vi "Style LED Blinking.vi"() -> ()   [LabVIEW 2015]
uses:
  <vilib>/Analysis/NI_AALBase.lvlib
panel:
  out "Boolean 8":bool
  out ".not. x?":bool
  in  "Magic Nmae Disply":bool
  in  "String":string
  out "concatenated string":string
  in  "Tab Control 2":enum32{"Page 1", "Page 2"}(tab)
  in  "Boolean":bool
  in  "Boolean 2":bool
  in  "Boolean 3":bool
  in  "Boolean 4":bool
  in  "Boolean 5":bool
  in  "Boolean 6":bool
  in  "duration":dbl
  in  "Tab Control":enum32{"Page 1", "Page 2"}(tab)
  out "Array":bool[][](array[boolean])
  in  "Time_1":dbl(knob) scale=0.0..1000.0
  out "Array 2":bool[][](array[boolean])
  in  "Control Statement":bool
  out "Array 3":bool[][](array[boolean])
  in  "?":u32(knob) scale=0.0..1000.0
  out "Array 5":bool[][](array[boolean])
  in  "Time_3":u32(knob) scale=0.0..1000.0
  out "Array 4":bool[][](array[boolean])
  out "Array 6":bool[][](array[boolean])
  # "Programming Happy Dussehra"
  # "Make Own Tune Press Button to PLAY"
  # "Time_2"
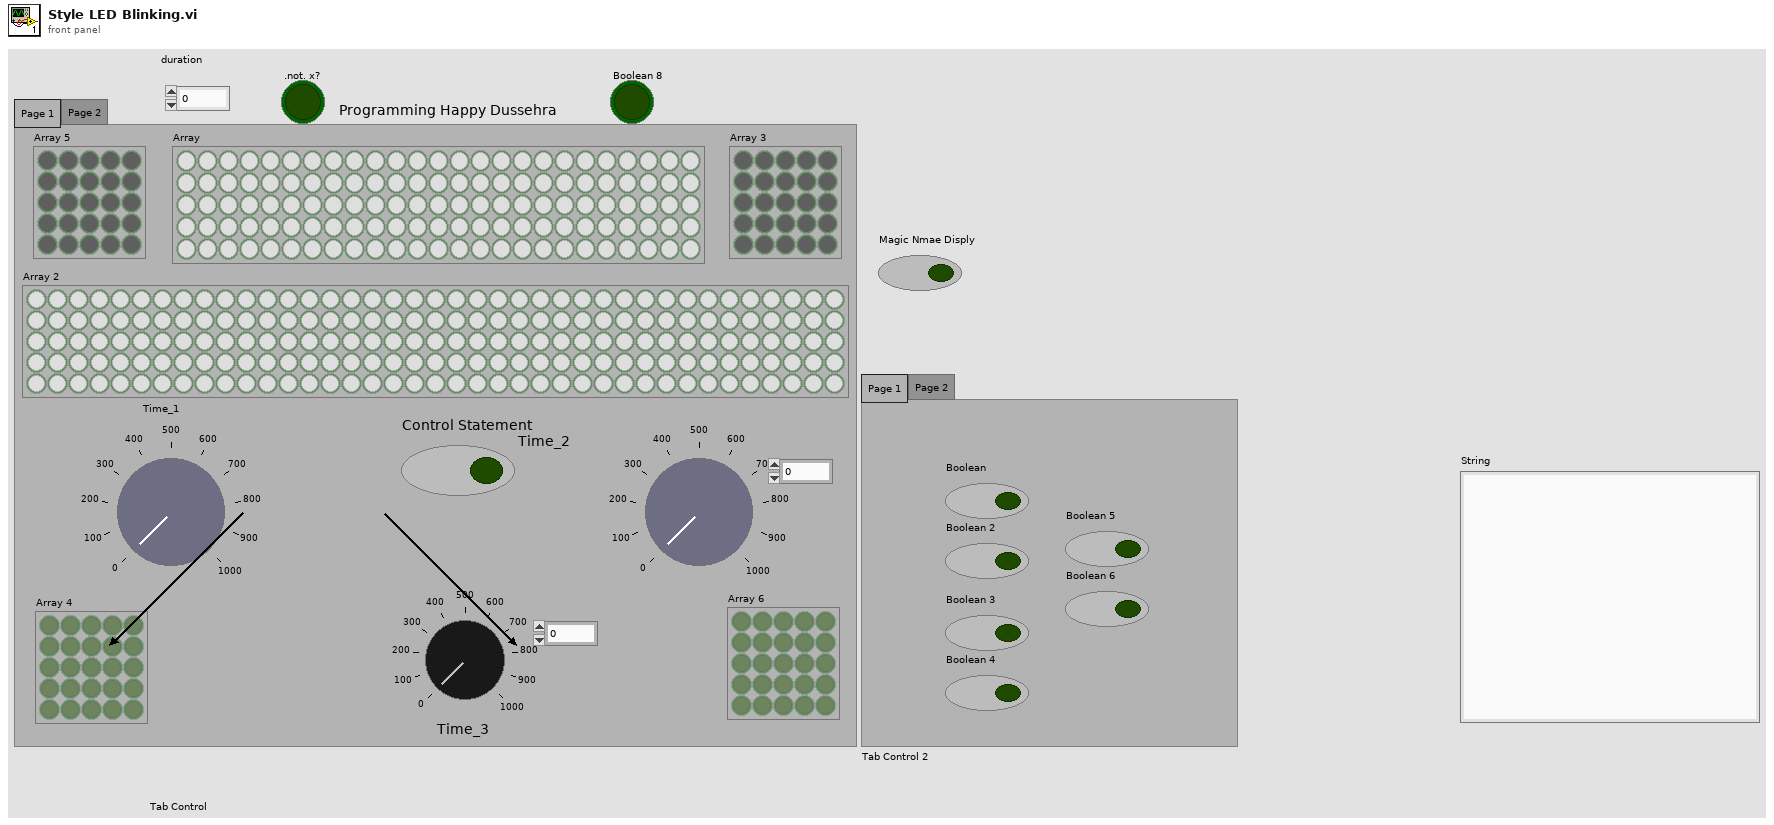
[diagram p1: front panel]
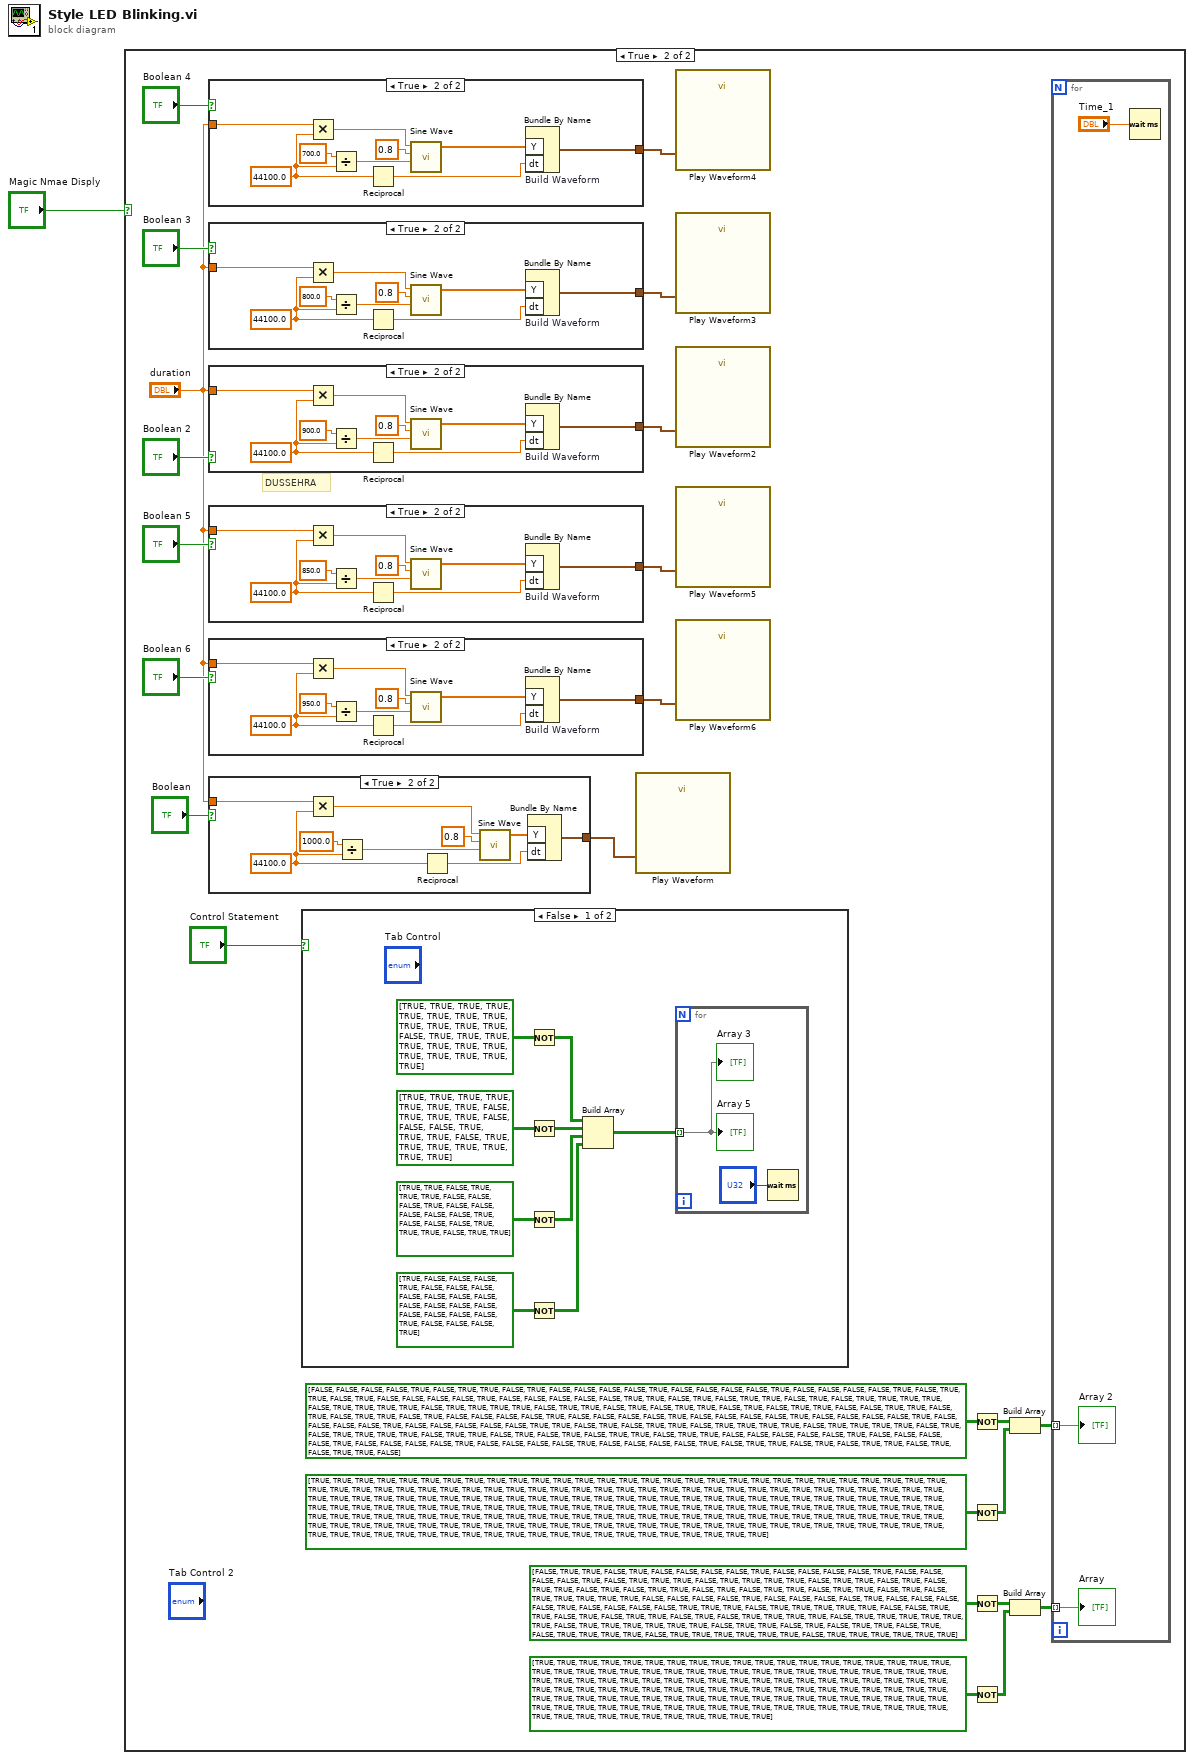
[diagram p0: block diagram]
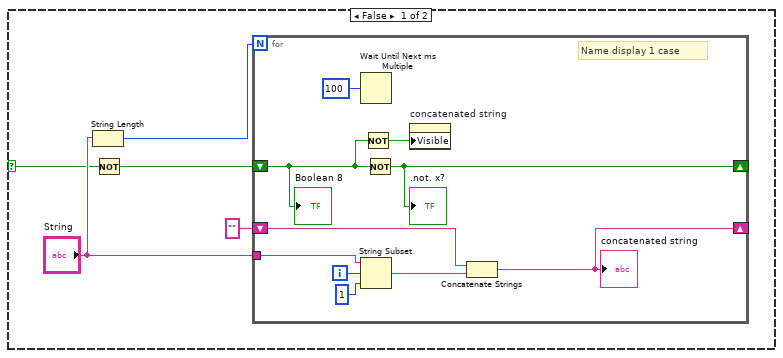
[diagram p2: hidden frame]
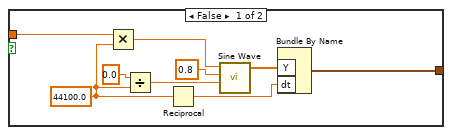
[diagram p3: hidden frame]
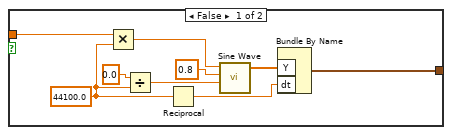
[diagram p4: hidden frame]
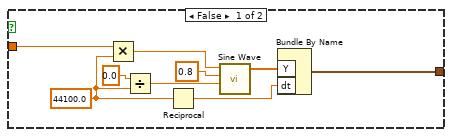
[diagram p5: hidden frame]
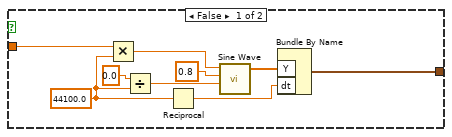
[diagram p6: hidden frame]
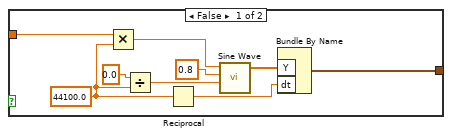
[diagram p7: hidden frame]
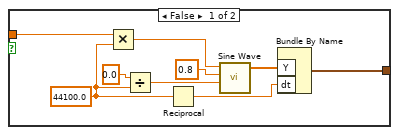
[diagram p8: hidden frame]
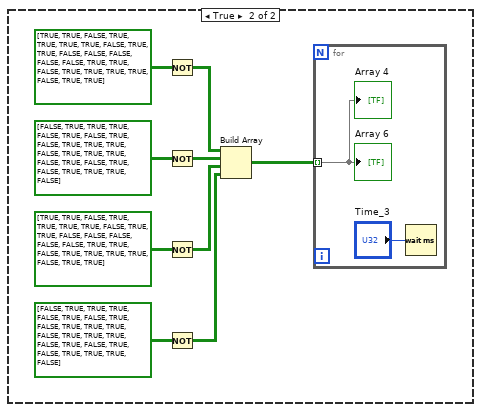
[diagram p9: hidden frame]
diagram:
  n1 = case shown="True" "Magic Nmae Disply" {
    selector: "Magic Nmae Disply" -> [w3 _]
    frame False {
      n2 = String Length(string="String") -> (length=w4:i32)
      n3 = Not(x=w3) -> (.not. x?=w2:bool)
      n4 = for {
        N: w4 -> [_]
        tunnel: "String" -> [w16]
        shift-right: [w12] -> _
        shift-left: "" -> [w11]
        shift-right: [w9] -> _
        shift-left: w2 -> [w7]
        i -> [w15]
        # "Name display 1 case"
        n5 = Wait Until Next ms Multiple(millisecond multiple=u32 100) -> ()  [unwired: 1 out]
        n6 = String Subset(string=w16, offset (0)=w15, length (rest)=1 ("length (rest)")) -> (substring=w13:string)
        n7 = Not(x=w7) -> (.not. x?=w8:bool)
        n8 = Not(x=w7) -> (.not. x?=w9:bool)
        ".not. x?" <- w9
        n9 = property on="concatenated string" class="Str"("Visible"=w8) -> ()  [unwired: 2 in, 2 out]
        n10 = Concatenate Strings "Concatenate Strings"(w11, w13) -> (w12:string)
        "concatenated string" <- w12
        "Boolean 8" <- w7
      }
    }
    frame True {
      # "DUSSEHRA"
      n11 = case shown="True" "Boolean 4" {
        tunnel: "duration" -> [w78 w88]
        tunnel: [w77 w87] -> w23
        frame False {
          w83 = 44100.0 ("fs(HZ) 3")
          n12 = Multiply(x=w78, y=w83) -> (x*y=w80:dbl)
          n13 = Divide(x=0.0 ("f(HZ) 2"), y=w83) -> (x/y=w81:dbl)
          n14 = Reciprocal(x=w83) -> (1/x=w84:dbl)
          n15 = call <vilib>:"Sine Wave.vi"("samples"=w80, "amplitude"=0.8, "frequency"=w81) -> ("sine wave"=w85:dbl[])  [unwired: 2 in, 2 out]
          n16 = Bundle By Name("Y"=w85, "dt"=w84) -> (w77:waveform(dbl))  [unwired: 1 in]
        }
        frame True {
          w92 = 44100.0 ("fs(HZ) 3")
          n17 = Multiply(x=w88, y=w92) -> (x*y=w89:dbl)
          n18 = Divide(x=700.0 ("f(HZ) 2"), y=w92) -> (x/y=w90:dbl)
          n19 = Reciprocal(x=w92) -> (1/x=w93:dbl)
          n20 = call <vilib>:"Sine Wave.vi"("samples"=w89, "amplitude"=0.8, "frequency"=w90) -> ("sine wave"=w94:dbl[])  [unwired: 2 in, 2 out]
          n21 = Bundle By Name "Build Waveform"("Y"=w94, "dt"=w93) -> (w87:waveform(dbl))  [unwired: 1 in]
        }
      }
      n22 = case shown="True" "Boolean 3" {
        tunnel: "duration" -> [w96 w106]
        tunnel: [w95 w105] -> w25
        frame False {
          w101 = 44100.0 ("fs(HZ) 3")
          n23 = Multiply(x=w96, y=w101) -> (x*y=w98:dbl)
          n24 = Divide(x=0.0 ("f(HZ) 2"), y=w101) -> (x/y=w99:dbl)
          n25 = Reciprocal(x=w101) -> (1/x=w102:dbl)
          n26 = call <vilib>:"Sine Wave.vi"("samples"=w98, "amplitude"=0.8, "frequency"=w99) -> ("sine wave"=w103:dbl[])  [unwired: 2 in, 2 out]
          n27 = Bundle By Name("Y"=w103, "dt"=w102) -> (w95:waveform(dbl))  [unwired: 1 in]
        }
        frame True {
          w110 = 44100.0 ("fs(HZ) 3")
          n28 = Multiply(x=w106, y=w110) -> (x*y=w107:dbl)
          n29 = Divide(x=800.0 ("f(HZ) 2"), y=w110) -> (x/y=w108:dbl)
          n30 = Reciprocal(x=w110) -> (1/x=w111:dbl)
          n31 = call <vilib>:"Sine Wave.vi"("samples"=w107, "amplitude"=0.8, "frequency"=w108) -> ("sine wave"=w112:dbl[])  [unwired: 2 in, 2 out]
          n32 = Bundle By Name "Build Waveform"("Y"=w112, "dt"=w111) -> (w105:waveform(dbl))  [unwired: 1 in]
        }
      }
      n33 = case shown="True" "Boolean 2" {
        tunnel: "duration" -> [w114 w124]
        tunnel: [w113 w123] -> w27
        frame False {
          w119 = 44100.0 ("fs(HZ) 3")
          n34 = Multiply(x=w114, y=w119) -> (x*y=w116:dbl)
          n35 = Divide(x=0.0 ("f(HZ) 2"), y=w119) -> (x/y=w117:dbl)
          n36 = Reciprocal(x=w119) -> (1/x=w120:dbl)
          n37 = call <vilib>:"Sine Wave.vi"("samples"=w116, "amplitude"=0.8, "frequency"=w117) -> ("sine wave"=w121:dbl[])  [unwired: 2 in, 2 out]
          n38 = Bundle By Name("Y"=w121, "dt"=w120) -> (w113:waveform(dbl))  [unwired: 1 in]
        }
        frame True {
          w128 = 44100.0 ("fs(HZ) 3")
          n39 = Multiply(x=w124, y=w128) -> (x*y=w125:dbl)
          n40 = Divide(x=900.0 ("f(HZ) 2"), y=w128) -> (x/y=w126:dbl)
          n41 = Reciprocal(x=w128) -> (1/x=w129:dbl)
          n42 = call <vilib>:"Sine Wave.vi"("samples"=w125, "amplitude"=0.8, "frequency"=w126) -> ("sine wave"=w130:dbl[])  [unwired: 2 in, 2 out]
          n43 = Bundle By Name "Build Waveform"("Y"=w130, "dt"=w129) -> (w123:waveform(dbl))  [unwired: 1 in]
        }
      }
      n44 = case shown="True" "Boolean 5" {
        tunnel: "duration" -> [w60 w70]
        tunnel: [w59 w69] -> w21
        frame False {
          w65 = 44100.0 ("fs(HZ) 3")
          n45 = Multiply(x=w60, y=w65) -> (x*y=w62:dbl)
          n46 = Divide(x=0.0 ("f(HZ) 2"), y=w65) -> (x/y=w63:dbl)
          n47 = Reciprocal(x=w65) -> (1/x=w66:dbl)
          n48 = call <vilib>:"Sine Wave.vi"("samples"=w62, "amplitude"=0.8, "frequency"=w63) -> ("sine wave"=w67:dbl[])  [unwired: 2 in, 2 out]
          n49 = Bundle By Name("Y"=w67, "dt"=w66) -> (w59:waveform(dbl))  [unwired: 1 in]
        }
        frame True {
          w74 = 44100.0 ("fs(HZ) 3")
          n50 = Multiply(x=w70, y=w74) -> (x*y=w71:dbl)
          n51 = Divide(x=850.0 ("f(HZ) 2"), y=w74) -> (x/y=w72:dbl)
          n52 = Reciprocal(x=w74) -> (1/x=w75:dbl)
          n53 = call <vilib>:"Sine Wave.vi"("samples"=w71, "amplitude"=0.8, "frequency"=w72) -> ("sine wave"=w76:dbl[])  [unwired: 2 in, 2 out]
          n54 = Bundle By Name "Build Waveform"("Y"=w76, "dt"=w75) -> (w69:waveform(dbl))  [unwired: 1 in]
        }
      }
      n55 = case shown="True" "Boolean 6" {
        tunnel: "duration" -> [w42 w52]
        tunnel: [w41 w51] -> w19
        frame False {
          w47 = 44100.0 ("fs(HZ) 3")
          n56 = Multiply(x=w42, y=w47) -> (x*y=w44:dbl)
          n57 = Divide(x=0.0 ("f(HZ) 2"), y=w47) -> (x/y=w45:dbl)
          n58 = Reciprocal(x=w47) -> (1/x=w48:dbl)
          n59 = call <vilib>:"Sine Wave.vi"("samples"=w44, "amplitude"=0.8, "frequency"=w45) -> ("sine wave"=w49:dbl[])  [unwired: 2 in, 2 out]
          n60 = Bundle By Name("Y"=w49, "dt"=w48) -> (w41:waveform(dbl))  [unwired: 1 in]
        }
        frame True {
          w56 = 44100.0 ("fs(HZ) 3")
          n61 = Multiply(x=w52, y=w56) -> (x*y=w53:dbl)
          n62 = Divide(x=950.0 ("f(HZ) 2"), y=w56) -> (x/y=w54:dbl)
          n63 = Reciprocal(x=w56) -> (1/x=w57:dbl)
          n64 = call <vilib>:"Sine Wave.vi"("samples"=w53, "amplitude"=0.8, "frequency"=w54) -> ("sine wave"=w58:dbl[])  [unwired: 2 in, 2 out]
          n65 = Bundle By Name "Build Waveform"("Y"=w58, "dt"=w57) -> (w51:waveform(dbl))  [unwired: 1 in]
        }
      }
      n66 = case shown="True" "Boolean" {
        tunnel: "duration" -> [w132 w142]
        tunnel: [w131 w141] -> w17
        frame False {
          w137 = 44100.0 ("fs(HZ) 3")
          n67 = Multiply(x=w132, y=w137) -> (x*y=w134:dbl)
          n68 = Divide(x=0.0 ("f(HZ) 2"), y=w137) -> (x/y=w135:dbl)
          n69 = Reciprocal(x=w137) -> (1/x=w138:dbl)
          n70 = call <vilib>:"Sine Wave.vi"("samples"=w134, "amplitude"=0.8, "frequency"=w135) -> ("sine wave"=w139:dbl[])  [unwired: 2 in, 2 out]
          n71 = Bundle By Name("Y"=w139, "dt"=w138) -> (w131:waveform(dbl))  [unwired: 1 in]
        }
        frame True {
          w146 = 44100.0 ("fs(HZ) 3")
          n72 = Multiply(x=w142, y=w146) -> (x*y=w143:dbl)
          n73 = Divide(x=1000.0 ("f(HZ) 2"), y=w146) -> (x/y=w144:dbl)
          n74 = Reciprocal(x=w146) -> (1/x=w147:dbl)
          n75 = call <vilib>:"Sine Wave.vi"("samples"=w143, "amplitude"=0.8, "frequency"=w144) -> ("sine wave"=w148:dbl[])  [unwired: 2 in, 2 out]
          n76 = Bundle By Name("Y"=w148, "dt"=w147) -> (w141:waveform(dbl))  [unwired: 1 in]
        }
      }
      n77 = case shown="False" "Control Statement" {
        frame False {
          n78 = Not(x=bool[][] [[TRUE, TRUE, TRUE, TRUE, TRUE], [TRUE, TRUE, TRUE, TRUE, TRUE], [TRUE, TRUE, FALSE, TRUE, TRUE], [TRUE, TRUE, TRUE, TRUE, TRUE], [TRUE, TRUE, TRUE, TRUE, TRUE]]) -> (.not. x?=w153:bool[][])
          n79 = Not(x=bool[][] [[TRUE, TRUE, TRUE, TRUE, TRUE], [TRUE, TRUE, FALSE, TRUE, TRUE], [TRUE, FALSE, FALSE, FALSE, TRUE], [TRUE, TRUE, FALSE, TRUE, TRUE], [TRUE, TRUE, TRUE, TRUE, TRUE]]) -> (.not. x?=w152:bool[][])
          n80 = Not(x=bool[][] [[TRUE, TRUE, FALSE, TRUE, TRUE], [TRUE, FALSE, FALSE, FALSE, TRUE], [FALSE, FALSE, FALSE, FALSE, FALSE], [TRUE, FALSE, FALSE, FALSE, TRUE], [TRUE, TRUE, FALSE, TRUE, TRUE]]) -> (.not. x?=w151:bool[][])
          n81 = Not(x=bool[][] [[TRUE, FALSE, FALSE, FALSE, TRUE], [FALSE, FALSE, FALSE, FALSE, FALSE], [FALSE, FALSE, FALSE, FALSE, FALSE], [FALSE, FALSE, FALSE, FALSE, FALSE], [TRUE, FALSE, FALSE, FALSE, TRUE]]) -> (.not. x?=w150:bool[][])
          n82 = Build Array "Build Array"(w153, w152, w151, w150) -> (w149:bool[][][])
          n83 = for {
            tunnel: w149 -> [w158] mode=indexing
            n84 = Wait (ms)(milliseconds to wait="?") -> ()  [unwired: 1 out]
            "Array 3" <- w158
            "Array 5" <- w158
          }
        }
        frame True {
          n85 = Not(x=bool[][] [[TRUE, TRUE, FALSE, TRUE, TRUE], [TRUE, TRUE, FALSE, TRUE, TRUE], [FALSE, FALSE, FALSE, FALSE, FALSE], [TRUE, TRUE, FALSE, TRUE, TRUE], [TRUE, TRUE, FALSE, TRUE, TRUE]]) -> (.not. x?=w164:bool[][])
          n86 = Not(x=bool[][] [[FALSE, TRUE, TRUE, TRUE, FALSE], [TRUE, FALSE, TRUE, FALSE, TRUE], [TRUE, TRUE, FALSE, TRUE, TRUE], [TRUE, FALSE, TRUE, FALSE, TRUE], [FALSE, TRUE, TRUE, TRUE, FALSE]]) -> (.not. x?=w163:bool[][])
          n87 = Not(x=bool[][] [[TRUE, TRUE, FALSE, TRUE, TRUE], [TRUE, TRUE, FALSE, TRUE, TRUE], [FALSE, FALSE, FALSE, FALSE, FALSE], [TRUE, TRUE, FALSE, TRUE, TRUE], [TRUE, TRUE, FALSE, TRUE, TRUE]]) -> (.not. x?=w162:bool[][])
          n88 = Not(x=bool[][] [[FALSE, TRUE, TRUE, TRUE, FALSE], [TRUE, FALSE, TRUE, FALSE, TRUE], [TRUE, TRUE, FALSE, TRUE, TRUE], [TRUE, FALSE, TRUE, FALSE, TRUE], [FALSE, TRUE, TRUE, TRUE, FALSE]]) -> (.not. x?=w161:bool[][])
          n89 = Build Array "Build Array"(w164, w163, w162, w161) -> (w160:bool[][][])
          n90 = for {
            tunnel: w160 -> [w169] mode=indexing
            n91 = Wait (ms)(milliseconds to wait="Time_3") -> ()  [unwired: 1 out]
            "Array 4" <- w169
            "Array 6" <- w169
          }
        }
      }
      n92 = call "Play Waveform"("Data"=w17) -> ()  [unwired: 18 in, 1 out]
      n93 = call "Play Waveform4"("Data"=w23) -> ()  [unwired: 18 in, 1 out]
      n94 = call "Play Waveform3"("Data"=w25) -> ()  [unwired: 18 in, 1 out]
      n95 = call "Play Waveform2"("Data"=w27) -> ()  [unwired: 18 in, 1 out]
      n96 = call "Play Waveform5"("Data"=w21) -> ()  [unwired: 18 in, 1 out]
      n97 = call "Play Waveform6"("Data"=w19) -> ()  [unwired: 18 in, 1 out]
      n98 = Not(x=bool[][] [[FALSE, FALSE, FALSE, FALSE, TRUE, FALSE, TRUE, TRUE, FALSE, TRUE, FALSE, FALSE, FALSE, FALSE, TRUE, FALSE, FALSE, FALSE, FALSE, TRUE, FALSE, FALSE, FALSE, FALSE, TRUE, FALSE, TRUE, TRUE, FALSE, TRUE, FALSE, FALSE, FALSE, FALSE, TRUE, FALSE, FALSE, FALSE, FALSE], [FALSE, TRUE, TRUE, FALSE, TRUE, FALSE, TRUE, TRUE, FALSE, TRUE, FALSE, TRUE, TRUE, TRUE, TRUE, FALSE, TRUE, TRUE, TRUE, TRUE, FALSE, TRUE, TRUE, TRUE, TRUE, FALSE, TRUE, TRUE, FALSE, TRUE, FALSE, TRUE, TRUE, FALSE, TRUE, FALSE, TRUE, TRUE, FALSE], [FALSE, TRUE, TRUE, FALSE, TRUE, FALSE, TRUE, TRUE, FALSE, TRUE, FALSE, FALSE, FALSE, FALSE, TRUE, FALSE, FALSE, FALSE, FALSE, TRUE, FALSE, FALSE, FALSE, FALSE, TRUE, FALSE, FALSE, FALSE, FALSE, TRUE, FALSE, FALSE, FALSE, FALSE, TRUE, FALSE, FALSE, FALSE, FALSE], [FALSE, TRUE, TRUE, FALSE, TRUE, FALSE, TRUE, TRUE, FALSE, TRUE, TRUE, TRUE, TRUE, FALSE, TRUE, TRUE, TRUE, TRUE, FALSE, TRUE, FALSE, TRUE, TRUE, TRUE, TRUE, FALSE, TRUE, TRUE, FALSE, TRUE, FALSE, TRUE, FALSE, TRUE, TRUE, FALSE, TRUE, TRUE, FALSE], [FALSE, FALSE, FALSE, FALSE, TRUE, FALSE, FALSE, FALSE, FALSE, TRUE, FALSE, FALSE, FALSE, FALSE, TRUE, FALSE, FALSE, FALSE, FALSE, TRUE, FALSE, FALSE, FALSE, FALSE, TRUE, FALSE, TRUE, TRUE, FALSE, TRUE, FALSE, TRUE, TRUE, FALSE, TRUE, FALSE, TRUE, TRUE, FALSE]]) -> (.not. x?=w33:bool[][])
      n99 = Not(x=bool[][] [[TRUE, TRUE, TRUE, TRUE, TRUE, TRUE, TRUE, TRUE, TRUE, TRUE, TRUE, TRUE, TRUE, TRUE, TRUE, TRUE, TRUE, TRUE, TRUE, TRUE, TRUE, TRUE, TRUE, TRUE, TRUE, TRUE, TRUE, TRUE, TRUE, TRUE, TRUE, TRUE, TRUE, TRUE, TRUE, TRUE, TRUE, TRUE, TRUE], [TRUE, TRUE, TRUE, TRUE, TRUE, TRUE, TRUE, TRUE, TRUE, TRUE, TRUE, TRUE, TRUE, TRUE, TRUE, TRUE, TRUE, TRUE, TRUE, TRUE, TRUE, TRUE, TRUE, TRUE, TRUE, TRUE, TRUE, TRUE, TRUE, TRUE, TRUE, TRUE, TRUE, TRUE, TRUE, TRUE, TRUE, TRUE, TRUE], [TRUE, TRUE, TRUE, TRUE, TRUE, TRUE, TRUE, TRUE, TRUE, TRUE, TRUE, TRUE, TRUE, TRUE, TRUE, TRUE, TRUE, TRUE, TRUE, TRUE, TRUE, TRUE, TRUE, TRUE, TRUE, TRUE, TRUE, TRUE, TRUE, TRUE, TRUE, TRUE, TRUE, TRUE, TRUE, TRUE, TRUE, TRUE, TRUE], [TRUE, TRUE, TRUE, TRUE, TRUE, TRUE, TRUE, TRUE, TRUE, TRUE, TRUE, TRUE, TRUE, TRUE, TRUE, TRUE, TRUE, TRUE, TRUE, TRUE, TRUE, TRUE, TRUE, TRUE, TRUE, TRUE, TRUE, TRUE, TRUE, TRUE, TRUE, TRUE, TRUE, TRUE, TRUE, TRUE, TRUE, TRUE, TRUE], [TRUE, TRUE, TRUE, TRUE, TRUE, TRUE, TRUE, TRUE, TRUE, TRUE, TRUE, TRUE, TRUE, TRUE, TRUE, TRUE, TRUE, TRUE, TRUE, TRUE, TRUE, TRUE, TRUE, TRUE, TRUE, TRUE, TRUE, TRUE, TRUE, TRUE, TRUE, TRUE, TRUE, TRUE, TRUE, TRUE, TRUE, TRUE, TRUE]]) -> (.not. x?=w32:bool[][])
      n100 = Not(x=bool[][] [[FALSE, TRUE, TRUE, FALSE, TRUE, FALSE, FALSE, FALSE, FALSE, TRUE, FALSE, FALSE, FALSE, FALSE, TRUE, FALSE, FALSE, FALSE, FALSE, TRUE, FALSE, TRUE, TRUE, TRUE, FALSE, TRUE, TRUE, TRUE, TRUE], [FALSE, TRUE, TRUE, FALSE, TRUE, FALSE, TRUE, TRUE, FALSE, TRUE, FALSE, TRUE, TRUE, FALSE, TRUE, FALSE, TRUE, TRUE, FALSE, TRUE, TRUE, FALSE, TRUE, FALSE, TRUE, TRUE, TRUE, TRUE, TRUE], [FALSE, FALSE, FALSE, FALSE, TRUE, FALSE, FALSE, FALSE, FALSE, TRUE, FALSE, FALSE, FALSE, FALSE, TRUE, FALSE, FALSE, FALSE, FALSE, TRUE, TRUE, TRUE, FALSE, TRUE, TRUE, TRUE, TRUE, TRUE, FALSE], [FALSE, TRUE, TRUE, FALSE, TRUE, FALSE, TRUE, TRUE, FALSE, TRUE, FALSE, TRUE, TRUE, TRUE, TRUE, FALSE, TRUE, TRUE, TRUE, TRUE, TRUE, TRUE, FALSE, TRUE, TRUE, TRUE, TRUE, TRUE, TRUE], [FALSE, TRUE, TRUE, FALSE, TRUE, FALSE, TRUE, TRUE, FALSE, TRUE, FALSE, TRUE, TRUE, TRUE, TRUE, FALSE, TRUE, TRUE, TRUE, TRUE, TRUE, TRUE, FALSE, TRUE, TRUE, TRUE, TRUE, TRUE, TRUE]]) -> (.not. x?=w38:bool[][])
      n101 = Not(x=bool[][] [[TRUE, TRUE, TRUE, TRUE, TRUE, TRUE, TRUE, TRUE, TRUE, TRUE, TRUE, TRUE, TRUE, TRUE, TRUE, TRUE, TRUE, TRUE, TRUE, TRUE, TRUE, TRUE, TRUE, TRUE, TRUE], [TRUE, TRUE, TRUE, TRUE, TRUE, TRUE, TRUE, TRUE, TRUE, TRUE, TRUE, TRUE, TRUE, TRUE, TRUE, TRUE, TRUE, TRUE, TRUE, TRUE, TRUE, TRUE, TRUE, TRUE, TRUE], [TRUE, TRUE, TRUE, TRUE, TRUE, TRUE, TRUE, TRUE, TRUE, TRUE, TRUE, TRUE, TRUE, TRUE, TRUE, TRUE, TRUE, TRUE, TRUE, TRUE, TRUE, TRUE, TRUE, TRUE, TRUE], [TRUE, TRUE, TRUE, TRUE, TRUE, TRUE, TRUE, TRUE, TRUE, TRUE, TRUE, TRUE, TRUE, TRUE, TRUE, TRUE, TRUE, TRUE, TRUE, TRUE, TRUE, TRUE, TRUE, TRUE, TRUE], [TRUE, TRUE, TRUE, TRUE, TRUE, TRUE, TRUE, TRUE, TRUE, TRUE, TRUE, TRUE, TRUE, TRUE, TRUE, TRUE, TRUE, TRUE, TRUE, TRUE, TRUE, TRUE, TRUE, TRUE, TRUE]]) -> (.not. x?=w36:bool[][])
      n102 = Build Array(w33, w32) -> (w31:bool[][][])
      n103 = Build Array(w38, w36) -> (w40:bool[][][])
      n104 = for {
        tunnel: w40 -> [w172] mode=indexing
        tunnel: w31 -> [w171] mode=indexing
        n105 = Wait (ms)(milliseconds to wait="Time_1") -> ()  [unwired: 1 out]
        "Array" <- w172
        "Array 2" <- w171
      }
    }
  }
